vi "NNPC_Init(Train).vi"(4 "PCore_Device":T1, 6 "Dataset_Stats":T4={"means"={"R"=0.66, "G"=0.59, "B"=0.44}, "vars"={"R"=0.66, "G"=0.59, "B"=0.44}, "DS_Size"=0} {"vars"."R" format="%#_3g"; "vars"."G" format="%#_3g"; "vars"."B" format="%#_3g"; "means"."R" format="%#_3g"; "means"."G" format="%#_3g"; "means"."B" format="%#_3g"}, 7 "NN_Paths":T2={"CFG"=path "D:/Ngene/Projects_SVN/DeepLTK/R_and_D/2024_02_01_Patchcore/LabVIEW/NN_Models/PCore_L2L3_Concat_224x224/wrn/wrn_net_cfg_24_08_02__10_26_58.cfg", "BIN"=path "D:/Ngene/Projects_SVN/DeepLTK/R_and_D/2024_02_01_Patchcore/LabVIEW/NN_Models/PCore_L2L3_Concat_224x224/wrn/wrn_weights_24_08_02__10_26_58.bin"}, 8 "error in (no error)":errorcluster, 9 "Coreset_Params":T25={"Sampling_Ratio"=0.1, "Startd_idx"=3, "Random_Proj?"=TRUE, "Rnd. Proj. Params"={"Proj._Dim."=-1, "Epsilon"=0.9, "Seed"=42}}, 10 "PatchCore_Init_CFG":T23={"BackBone"=enum."WRN_50_2_L2L3", "Out_Layers_Names"=["L2", "L3"], "Patch_Size"=3}, 11 "NNFE_Custom_CFG":T28={"Input3D_Custom_Dims"={"C"=-1, "H"=-1, "W"=-1}, "mBatch"=1, "NN_Device"=enum."CPU"}) -> (0 "error out":errorcluster, 3 "PCore_Instance out":T3={"Dataset_Stats"={"means"={"R"=0.66, "G"=0.59, "B"=0.44}, "vars"={"R"=0.66, "G"=0.59, "B"=0.44}, "DS_Size"=0}, "NN"={"Name"="wrn", "No of Layers"=63, "mBatch"=1, "Layers"=[refnum, refnum, refnum, refnum, refnum, refnum, refnum, refnum, refnum, refnum, refnum, refnum, refnum, refnum, refnum, refnum, refnum, refnum, refnum, refnum, refnum, refnum, refnum, refnum, refnum, refnum, refnum, refnum, refnum, refnum, refnum, refnum, refnum, refnum, refnum, refnum, refnum, refnum, refnum, refnum, refnum, refnum, refnum, refnum, refnum, refnum, refnum, refnum, refnum, refnum, refnum, refnum, refnum, refnum, refnum, refnum, refnum, refnum, refnum, refnum, refnum, refnum, refnum], "Dimty"=enum."In3D_Out3D", "Dims_In"={"C"=3, "H"=224, "W"=224}, "Dims_Out"={"C"=302, "H"=28, "W"=28}, "Working_Dir"=path "D:/Ngene/Projects_SVN/DeepLTK/R_and_D/2024_02_01_Patchcore/LabVIEW/PatchCore_v5.0/working/wrn", "Train?"=FALSE, "Train_Params"={"Optimizer"=enum."SGD", "Beta_1"=0.999, "Beta_2"=0.999, "Weight Decay(L1)"=0.0, "Weight Decay(L2)"=0.0, "Data_Sampling"=enum."Random"}, "LR_Update_Policy"={"Policy_Type"=enum."Manual", "LR0"=0.0, "k"=0.0, "WarmUp_Policy"=enum."Step", "WarmUp_Iter"=100, "WarmUp_Ratio"=10.0}, "Session Data"={"Epochs"=0.0, "Tot_Iter"=1, "LR"=0.0, "LR_iter"=1}, "Ground_truth"={"Y"=variant(refnum<data-value> refnum)}, "NNg_hdls"={"cudnn"=2143106709504, "cublas"=2177817002560, "stream"=2141212075440, "curand"=2143055681792}, "NN_Device"=enum."GPU", "GPU Id"=0, "Labels"=["tench", "goldfish", "great white shark", "tiger shark", "hammerhead", "electric ray", "stingray", "cock", "hen", "ostrich", "brambling", "goldfinch", "house finch", "junco", "indigo bunting", "robin", "bulbul", "jay", "magpie", "chickadee", "water ouzel", "kite", "bald eagle", "vulture", "great grey owl", "European fire salamander", "common newt", "eft", "spotted salamander", "axolotl", "bullfrog", "tree frog", "tailed frog", "loggerhead", "leatherback turtle", "mud turtle", "terrapin", "box turtle", "banded gecko", "common iguana", "American chameleon", "whiptail", "agama", "frilled lizard", "alligator lizard", "Gila monster", "green lizard", "African chameleon", "Komodo dragon", "African crocodile", "American alligator", "triceratops", "thunder snake", "ringneck snake", "hognose snake", "green snake", "king snake", "garter snake", "water snake", "vine snake", "night snake", "boa constrictor", "rock python", "Indian cobra", "green mamba", "sea snake", "horned viper", "diamondback", "sidewinder", "trilobite", "harvestman", "scorpion", "black and gold garden spider", "barn spider", "garden spider", "black widow", "tarantula", "wolf spider", "tick", "centipede", "black grouse", "ptarmigan", "ruffed grouse", "prairie chicken", "peacock", "quail", "partridge", "African grey", "macaw", "sulphur-crested cockatoo", "lorikeet", "coucal", "bee eater", "hornbill", "hummingbird", "jacamar", "toucan", "drake", "red-breasted merganser", "goose", "black swan", "tusker", "echidna", "platypus", "wallaby", "koala", "wombat", "jellyfish", "sea anemone", "brain coral", "flatworm", "nematode", "conch", "snail", "slug", "sea slug", "chiton", "chambered nautilus", "Dungeness crab", "rock crab", "fiddler crab", "king crab", "American lobster", "spiny lobster", "crayfish", "hermit crab", "isopod", "white stork", "black stork", "spoonbill", "flamingo", "little blue heron", "American egret", "bittern", "crane", "limpkin", "European gallinule", "American coot", "bustard", "ruddy turnstone", "red-backed sandpiper", "redshank", "dowitcher", "oystercatcher", "pelican", "king penguin", "albatross", "grey whale", "killer whale", "dugong", "sea lion", "Chihuahua", "Japanese spaniel", "Maltese dog", "Pekinese", "Shih-Tzu", "Blenheim spaniel", "papillon", "toy terrier", "Rhodesian ridgeback", "Afghan hound", "basset", "beagle", "bloodhound", "bluetick", "black-and-tan coonhound", "Walker hound", "English foxhound", "redbone", "borzoi", "Irish wolfhound", "Italian greyhound", "whippet", "Ibizan hound", "Norwegian elkhound", "otterhound", "Saluki", "Scottish deerhound", "Weimaraner", "Staffordshire bullterrier", "American Staffordshire terrier", "Bedlington terrier", "Border terrier", "Kerry blue terrier", "Irish terrier", "Norfolk terrier", "Norwich terrier", "Yorkshire terrier", "wire-haired fox terrier", "Lakeland terrier", "Sealyham terrier", "Airedale", "cairn", "Australian terrier", "Dandie Dinmont", "Boston bull", "miniature schnauzer", "giant schnauzer", "standard schnauzer", "Scotch terrier", "Tibetan terrier", "silky terrier", "soft-coated wheaten terrier", "West Highland white terrier", "Lhasa", "flat-coated retriever", "curly-coated retriever", "golden retriever", "Labrador retriever", "Chesapeake Bay retriever", "German short-haired pointer", "vizsla", "English setter", "Irish setter", "Gordon setter", "Brittany spaniel", "clumber", "English springer", "Welsh springer spaniel", "cocker spaniel", "Sussex spaniel", "Irish water spaniel", "kuvasz", "schipperke", "groenendael", "malinois", "briard", "kelpie", "komondor", "Old English sheepdog", "Shetland sheepdog", "collie", "Border collie", "Bouvier des Flandres", "Rottweiler", "German shepherd", "Doberman", "miniature pinscher", "Greater Swiss Mountain dog", "Bernese mountain dog", "Appenzeller", "EntleBucher", "boxer", "bull mastiff", "Tibetan mastiff", "French bulldog", "Great Dane", "Saint Bernard", "Eskimo dog", "malamute", "Siberian husky", "dalmatian", "affenpinscher", "basenji", "pug", "Leonberg", "Newfoundland", "Great Pyrenees", "Samoyed", "Pomeranian", "chow", "keeshond", "Brabancon griffon", "Pembroke", "Cardigan", "toy poodle", "miniature poodle", "standard poodle", "Mexican hairless", "timber wolf", "white wolf", "red wolf", "coyote", "dingo", "dhole", "African hunting dog", "hyena", "red fox", "kit fox", "Arctic fox", "grey fox", "tabby", "tiger cat", "Persian cat", "Siamese cat", "Egyptian cat", "cougar", "lynx", "leopard", "snow leopard", "jaguar", "lion", "tiger", "cheetah", "brown bear", "American black bear", "ice bear", "sloth bear", "mongoose", "meerkat", "tiger beetle", "ladybug", "ground beetle", "long-horned beetle", "leaf beetle", "dung beetle", "rhinoceros beetle", "weevil", "fly", "bee", "ant", "grasshopper", "cricket", "walking stick", "cockroach", "mantis", "cicada", "leafhopper", "lacewing", "dragonfly", "damselfly", "admiral", "ringlet", "monarch", "cabbage butterfly", "sulphur butterfly", "lycaenid", "starfish", "sea urchin", "sea cucumber", "wood rabbit", "hare", "Angora", "hamster", "porcupine", "fox squirrel", "marmot", "beaver", "guinea pig", "sorrel", "zebra", "hog", "wild boar", "warthog", "hippopotamus", "ox", "water buffalo", "bison", "ram", "bighorn", "ibex", "hartebeest", "impala", "gazelle", "Arabian camel", "llama", "weasel", "mink", "polecat", "black-footed ferret", "otter", "skunk", "badger", "armadillo", "three-toed sloth", "orangutan", "gorilla", "chimpanzee", "gibbon", "siamang", "guenon", "patas", "baboon", "macaque", "langur", "colobus", "proboscis monkey", "marmoset", "capuchin", "howler monkey", "titi", "spider monkey", "squirrel monkey", "Madagascar cat", "indri", "Indian elephant", "African elephant", "lesser panda", "giant panda", "barracouta", "eel", "coho", "rock beauty", "anemone fish", "sturgeon", "gar", "lionfish", "puffer", "abacus", "abaya", "academic gown", "accordion", "acoustic guitar", "aircraft carrier", "airliner", "airship", "altar", "ambulance", "amphibian", "analog clock", "apiary", "apron", "ashcan", "assault rifle", "backpack", "bakery", "balance beam", "balloon", "ballpoint", "Band Aid", "banjo", "bannister", "barbell", "barber chair", "barbershop", "barn", "barometer", "barrel", "barrow", "baseball", "basketball", "bassinet", "bassoon", "bathing cap", "bath towel", "bathtub", "beach wagon", "beacon", "beaker", "bearskin", "beer bottle", "beer glass", "bell cote", "bib", "bicycle-built-for-two", "bikini", "binder", "binoculars", "birdhouse", "boathouse", "bobsled", "bolo tie", "bonnet", "bookcase", "bookshop", "bottlecap", "bow", "bow tie", "brass", "brassiere", "breakwater", "breastplate", "broom", "bucket", "buckle", "bulletproof vest", "bullet train", "butcher shop", "cab", "caldron", "candle", "cannon", "canoe", "can opener", "cardigan", "car mirror", "carousel", "carpenter's kit", "carton", "car wheel", "cash machine", "cassette", "cassette player", "castle", "catamaran", "CD player", "cello", "cellular telephone", "chain", "chainlink fence", "chain mail", "chain saw", "chest", "chiffonier", "chime", "china cabinet", "Christmas stocking", "church", "cinema", "cleaver", "cliff dwelling", "cloak", "clog", "cocktail shaker", "coffee mug", "coffeepot", "coil", "combination lock", "computer keyboard", "confectionery", "container ship", "convertible", "corkscrew", "cornet", "cowboy boot", "cowboy hat", "cradle", "crane", "crash helmet", "crate", "crib", "Crock Pot", "croquet ball", "crutch", "cuirass", "dam", "desk", "desktop computer", "dial telephone", "diaper", "digital clock", "digital watch", "dining table", "dishrag", "dishwasher", "disk brake", "dock", "dogsled", "dome", "doormat", "drilling platform", "drum", "drumstick", "dumbbell", "Dutch oven", "electric fan", "electric guitar", "electric locomotive", "entertainment center", "envelope", "espresso maker", "face powder", "feather boa", "file", "fireboat", "fire engine", "fire screen", "flagpole", "flute", "folding chair", "football helmet", "forklift", "fountain", "fountain pen", "four-poster", "freight car", "French horn", "frying pan", "fur coat", "garbage truck", "gasmask", "gas pump", "goblet", "go-kart", "golf ball", "golfcart", "gondola", "gong", "gown", "grand piano", "greenhouse", "grille", "grocery store", "guillotine", "hair slide", "hair spray", "half track", "hammer", "hamper", "hand blower", "hand-held computer", "handkerchief", "hard disc", "harmonica", "harp", "harvester", "hatchet", "holster", "home theater", "honeycomb", "hook", "hoopskirt", "horizontal bar", "horse cart", "hourglass", "iPod", "iron", "jack-o'-lantern", "jean", "jeep", "jersey", "jigsaw puzzle", "jinrikisha", "joystick", "kimono", "knee pad", "knot", "lab coat", "ladle", "lampshade", "laptop", "lawn mower", "lens cap", "letter opener", "library", "lifeboat", "lighter", "limousine", "liner", "lipstick", "Loafer", "lotion", "loudspeaker", "loupe", "lumbermill", "magnetic compass", "mailbag", "mailbox", "maillot", "maillot", "manhole cover", "maraca", "marimba", "mask", "matchstick", "maypole", "maze", "measuring cup", "medicine chest", "megalith", "microphone", "microwave", "military uniform", "milk can", "minibus", "miniskirt", "minivan", "missile", "mitten", "mixing bowl", "mobile home", "Model T", "modem", "monastery", "monitor", "moped", "mortar", "mortarboard", "mosque", "mosquito net", "motor scooter", "mountain bike", "mountain tent", "mouse", "mousetrap", "moving van", "muzzle", "nail", "neck brace", "necklace", "nipple", "notebook", "obelisk", "oboe", "ocarina", "odometer", "oil filter", "organ", "oscilloscope", "overskirt", "oxcart", "oxygen mask", "packet", "paddle", "paddlewheel", "padlock", "paintbrush", "pajama", "palace", "panpipe", "paper towel", "parachute", "parallel bars", "park bench", "parking meter", "passenger car", "patio", "pay-phone", "pedestal", "pencil box", "pencil sharpener", "perfume", "Petri dish", "photocopier", "pick", "pickelhaube", "picket fence", "pickup", "pier", "piggy bank", "pill bottle", "pillow", "ping-pong ball", "pinwheel", "pirate", "pitcher", "plane", "planetarium", "plastic bag", "plate rack", "plow", "plunger", "Polaroid camera", "pole", "police van", "poncho", "pool table", "pop bottle", "pot", "potter's wheel", "power drill", "prayer rug", "printer", "prison", "projectile", "projector", "puck", "punching bag", "purse", "quill", "quilt", "racer", "racket", "radiator", "radio", "radio telescope", "rain barrel", "recreational vehicle", "reel", "reflex camera", "refrigerator", "remote control", "restaurant", "revolver", "rifle", "rocking chair", "rotisserie", "rubber eraser", "rugby ball", "rule", "running shoe", "safe", "safety pin", "saltshaker", "sandal", "sarong", "sax", "scabbard", "scale", "school bus", "schooner", "scoreboard", "screen", "screw", "screwdriver", "seat belt", "sewing machine", "shield", "shoe shop", "shoji", "shopping basket", "shopping cart", "shovel", "shower cap", "shower curtain", "ski", "ski mask", "sleeping bag", "slide rule", "sliding door", "slot", "snorkel", "snowmobile", "snowplow", "soap dispenser", "soccer ball", "sock", "solar dish", "sombrero", "soup bowl", "space bar", "space heater", "space shuttle", "spatula", "speedboat", "spider web", "spindle", "sports car", "spotlight", "stage", "steam locomotive", "steel arch bridge", "steel drum", "stethoscope", "stole", "stone wall", "stopwatch", "stove", "strainer", "streetcar", "stretcher", "studio couch", "stupa", "submarine", "suit", "sundial", "sunglass", "sunglasses", "sunscreen", "suspension bridge", "swab", "sweatshirt", "swimming trunks", "swing", "switch", "syringe", "table lamp", "tank", "tape player", "teapot", "teddy", "television", "tennis ball", "thatch", "theater curtain", "thimble", "thresher", "throne", "tile roof", "toaster", "tobacco shop", "toilet seat", "torch", "totem pole", "tow truck", "toyshop", "tractor", "trailer truck", "tray", "trench coat", "tricycle", "trimaran", "tripod", "triumphal arch", "trolleybus", "trombone", "tub", "turnstile", "typewriter keyboard", "umbrella", "unicycle", "upright", "vacuum", "vase", "vault", "velvet", "vending machine", "vestment", "viaduct", "violin", "volleyball", "waffle iron", "wall clock", "wallet", "wardrobe", "warplane", "washbasin", "washer", "water bottle", "water jug", "water tower", "whiskey jug", "whistle", "wig", "window screen", "window shade", "Windsor tie", "wine bottle", "wing", "wok", "wooden spoon", "wool", "worm fence", "wreck", "yawl", "yurt", "web site", "comic book", "crossword puzzle", "street sign", "traffic light", "book jacket", "menu", "plate", "guacamole", "consomme", "hot pot", "trifle", "ice cream", "ice lolly", "French loaf", "bagel", "pretzel", "cheeseburger", "hotdog", "mashed potato", "head cabbage", "broccoli", "cauliflower", "zucchini", "spaghetti squash", "acorn squash", "butternut squash", "cucumber", "artichoke", "bell pepper", "cardoon", "mushroom", "Granny Smith", "strawberry", "orange", "lemon", "fig", "pineapple", "banana", "jackfruit", "custard apple", "pomegranate", "hay", "carbonara", "chocolate sauce", "dough", "meat loaf", "pizza", "potpie", "burrito", "red wine", "espresso", "cup", "eggnog", "alp", "bubble", "cliff", "coral reef", "geyser", "lakeside", "promontory", "sandbar", "seashore", "valley", "volcano", "ballplayer", "groom", "scuba diver", "rapeseed", "daisy", "yellow lady's slipper", "corn", "acorn", "hip", "buckeye", "coral fungus", "agaric", "gyromitra", "stinkhorn", "earthstar", "hen-of-the-woods", "bolete", "ear", "toilet tissue"], "Receptive Field"=[{"V"=1, "H"=1}, {"V"=7, "H"=7}, {"V"=9, "H"=9}, {"V"=9, "H"=9}, {"V"=21, "H"=21}, {"V"=21, "H"=21}, {"V"=9, "H"=9}, {"V"=21, "H"=21}, {"V"=21, "H"=21}, {"V"=33, "H"=33}, {"V"=33, "H"=33}, {"V"=33, "H"=33}, {"V"=33, "H"=33}, {"V"=45, "H"=45}, {"V"=45, "H"=45}, {"V"=45, "H"=45}, {"V"=45, "H"=45}, {"V"=57, "H"=57}, {"V"=57, "H"=57}, {"V"=45, "H"=45}, {"V"=57, "H"=57}, {"V"=57, "H"=57}, {"V"=81, "H"=81}, {"V"=81, "H"=81}, {"V"=81, "H"=81}, {"V"=81, "H"=81}, {"V"=105, "H"=105}, {"V"=105, "H"=105}, {"V"=105, "H"=105}, {"V"=105, "H"=105}, {"V"=129, "H"=129}, {"V"=129, "H"=129}, {"V"=129, "H"=129}, {"V"=129, "H"=129}, {"V"=153, "H"=153}, {"V"=153, "H"=153}, {"V"=129, "H"=129}, {"V"=153, "H"=153}, {"V"=153, "H"=153}, {"V"=201, "H"=201}, {"V"=201, "H"=201}, {"V"=201, "H"=201}, {"V"=201, "H"=201}, {"V"=249, "H"=249}, {"V"=249, "H"=249}, {"V"=249, "H"=249}, {"V"=249, "H"=249}, {"V"=297, "H"=297}, {"V"=297, "H"=297}, {"V"=297, "H"=297}, {"V"=297, "H"=297}, {"V"=345, "H"=345}, {"V"=345, "H"=345}, {"V"=345, "H"=345}, {"V"=345, "H"=345}, {"V"=393, "H"=393}, {"V"=393, "H"=393}, {"V"=393, "H"=393}, {"V"=153, "H"=153}, {"V"=441, "H"=441}, {"V"=441, "H"=441}, {"V"=441, "H"=441}, {"V"=441, "H"=441}], "Loss_Type"=enum."MSE", "Loss_Cfg_Prms"=variant, "NNG_WS"={"NNG_WS_Mem"=refnum, "Max_WS_Size"=-1}}, "PCore_Device"=enum."GPU(CuLab)", "PatchCore_Init_CFG"={"BackBone"=enum."WRN_50_2_L2L3", "Out_Layers_Names"=[], "Patch_Size"=0}, "Coreset Params"={"Sampling_Ratio"=0.0, "Startd_idx"=0, "Random_Proj?"=FALSE, "Rnd. Proj. Params"={"Proj._Dim."=0, "Epsilon"=0.9, "Seed"=42}}, "MemBank_Data"={"MemBank"=variant, "MemBank Norm"=variant}} {"NN out"."LR_Update_Policy"."WarmUp_Ratio" min=1; "NN out"."LR_Update_Policy"."WarmUp_Iter" min=1; "NN out"."LR_Update_Policy"."LR0" format="%.7f"; "Dataset_Stats"."vars"."R" format="%#_3g"; "Dataset_Stats"."vars"."G" format="%#_3g"; "Dataset_Stats"."vars"."B" format="%#_3g"; "Dataset_Stats"."means"."R" format="%#_3g"; "Dataset_Stats"."means"."G" format="%#_3g"; "Dataset_Stats"."means"."B" format="%#_3g"}, 5 "dT":dbl)   [LabVIEW 2020]
uses:
  Controls/PatchCore_Init_CFG.ctl
  Controls/PatchCore_BackBone_Selector.ctl
  Controls/PatchCore_Init_Custom_NN_CFG.ctl
  <vilib>/Ngene/Deep Learning Toolkit/Toolkit/NN_Data/API/NN_Dims(C,H,W).ctl
  <vilib>/Ngene/Deep Learning Toolkit/Toolkit/NN_Network/Controls/NN_Device.ctl
  Controls/PatchCore_DS_Stats.ctl
  Controls/Image_Stats_RGB.ctl
  Controls/Coreset_Params.ctl
  Controls/Random_Projection_Coreset.ctl
  Controls/PatchCore_Instance.ctl
  <vilib>/Ngene/Deep Learning Toolkit/Toolkit/NN_Network/Controls/NN.ctl
  <vilib>/Ngene/Deep Learning Toolkit/Toolkit/NN_Layers/Controls/NN_Layer_ref.ctl
  <vilib>/Ngene/Deep Learning Toolkit/Toolkit/NN_Layers/Controls/NN_Layer.ctl
  <vilib>/Ngene/Deep Learning Toolkit/Toolkit/NN_Layers/Controls/NN_Layer_Type.ctl
  <vilib>/Ngene/Deep Learning Toolkit/Toolkit/NN_Layers/Controls/NN_Layer_Metrics.ctl
  <vilib>/Ngene/Deep Learning Toolkit/Toolkit/NNg/cuda/Controls/nng_cuda_handles.ctl
  <vilib>/Ngene/Deep Learning Toolkit/Toolkit/NN_Layers/Controls/NN_Layer_Dimty.ctl
  <vilib>/Ngene/Deep Learning Toolkit/Toolkit/NN_Layers/Controls/NN_Layer_RF_State.ctl
  <vilib>/Ngene/Deep Learning Toolkit/Toolkit/NN_Data/API/NN_Dims(V,H).ctl
  <vilib>/Ngene/Deep Learning Toolkit/Toolkit/NN_Network/Controls/NN_In_Out_Dim-ty.ctl
  <vilib>/Ngene/Deep Learning Toolkit/Toolkit/NN_Train/Controls/NN_Train_Params.ctl
  <vilib>/Ngene/Deep Learning Toolkit/Toolkit/NN_Train/Controls/NN_Train_Optimizer.ctl
  <vilib>/Ngene/Deep Learning Toolkit/Toolkit/NN_Train/Controls/NN_Train_Data_Sampling.ctl
  <vilib>/Ngene/Deep Learning Toolkit/Toolkit/NN_Train/Controls/NN_LR_Policy_Cfg.ctl
  <vilib>/Ngene/Deep Learning Toolkit/Toolkit/NN_Train/Controls/NN_LR_Policy_Type.ctl
  <vilib>/Ngene/Deep Learning Toolkit/Toolkit/NN_Train/Controls/NN_Train_Session_Data.ctl
  <vilib>/Ngene/Deep Learning Toolkit/Toolkit/NN_Data/Controls/NN_Ground_truth.ctl
  <vilib>/Ngene/Deep Learning Toolkit/Toolkit/NN_Train/Controls/NN_Loss_Type.ctl
  <vilib>/Ngene/Deep Learning Toolkit/Toolkit/NNg/Network/WS/Controls/NNG_WS.ctl
  <vilib>/Ngene/Deep Learning Toolkit/Toolkit/NNg/Network/WS/Controls/NNg_WS_Mem_DVR.ctl
  <vilib>/Ngene/Deep Learning Toolkit/Toolkit/NNg/cuda/Controls/cuda_Mem_desc.ctl
  Controls/PCore_Device.ctl
  Controls/MemBank_and_Norm_Variants.ctl
  Controls/NN_Paths.ctl
  edddb0eb-9e83-41dd-b3bf-18adf70eff0a.vi
  e3f785a9-3252-4081-a6fc-ec5b49997386.vi
  <vilib>/Utility/High Resolution Relative Seconds.vi
  <vilib>/Ngene/Deep Learning Toolkit/Toolkit/Deep_Learning_Toolkit_by_Ngene.lvlib
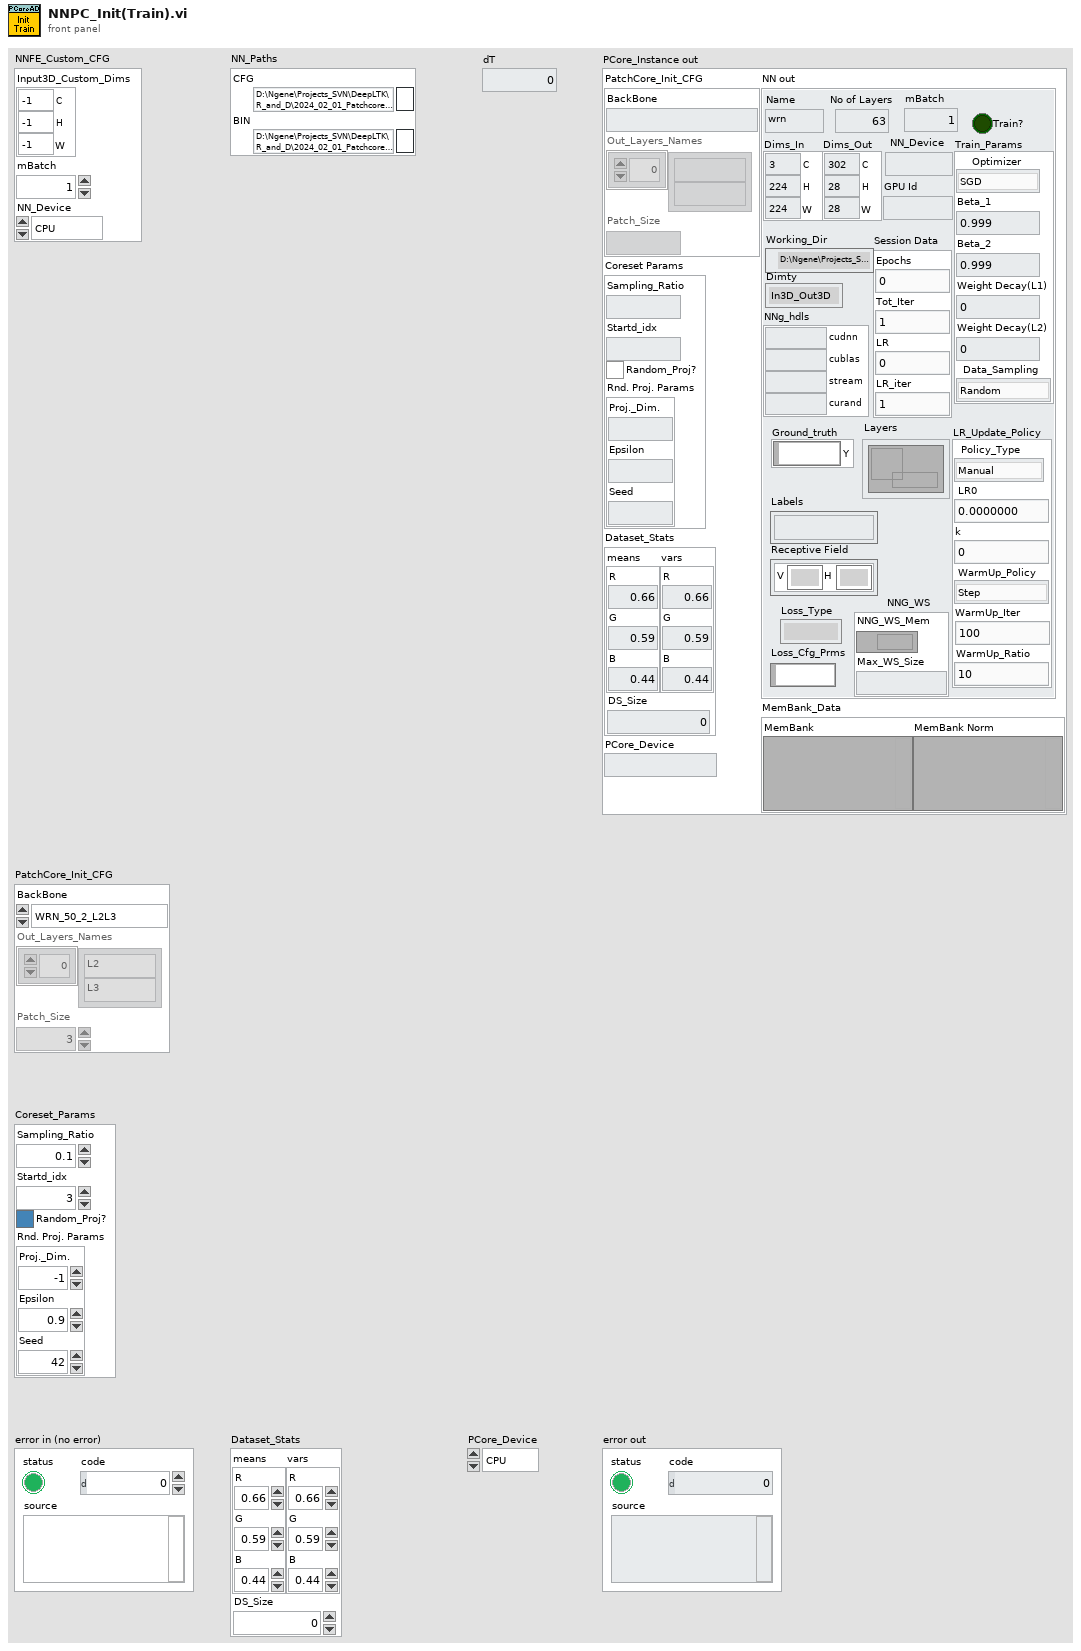
[diagram p1: front panel]
types:
  T1 = typedef "PCore_Device.ctl" = enum16{"CPU", "GPU(CuLab)"}
  T2 = typedef "NN_Paths.ctl" = cluster{"CFG":path, "BIN":path}
  T3 = typedef "PatchCore_Instance.ctl" = cluster{"Dataset_Stats":T4, "NN":T6, "PCore_Device":T1, "PatchCore_Init_CFG":T23, "Coreset Params":T25, "MemBank_Data":T27}
  T4 = typedef "PatchCore_DS_Stats.ctl" = cluster{"means":T5, "vars":T5, "DS_Size":i32}
  T5 = typedef "Image_Stats_RGB.ctl" = cluster{"R":sgl, "G":sgl, "B":sgl}
  T6 = typedef "Deep_Learning_Toolkit_by_Ngene.lvlib/NN.ctl" = cluster{"Name":string, "No of Layers":i32, "mBatch":i32, "Layers":T7[], "Dimty":T8, "Dims_In":T9, "Dims_Out":T9, "Working_Dir":path, "Train?":bool, "Train_Params":T10, "LR_Update_Policy":T13, "Session Data":T15, "Ground_truth":T16, "NNg_hdls":T17, "NN_Device":T18, "GPU Id":i32, "Labels":string[], "Receptive Field":T19[], "Loss_Type":T20, "Loss_Cfg_Prms":variant, "NNG_WS":T21}
  T7 = typedef "Deep_Learning_Toolkit_by_Ngene.lvlib/NN_Layer_ref.ctl" = refnum<data-value>
  T8 = typedef "Deep_Learning_Toolkit_by_Ngene.lvlib/NN_In_Out_Dim-ty.ctl" = enum8{"In1D_Out1D", "In3D_Out1D", "In3D_Out3D", "In3D_OutBBox"}
  T9 = typedef "Deep_Learning_Toolkit_by_Ngene.lvlib/NN_Dims(C,H,W).ctl" = cluster{"C":i32, "H":i32, "W":i32}
  T10 = typedef "Deep_Learning_Toolkit_by_Ngene.lvlib/NN_Train_Params.ctl" = cluster{"Optimizer":T11, "Beta_1":sgl, "Beta_2":sgl, "Weight Decay(L1)":sgl, "Weight Decay(L2)":sgl, "Data_Sampling":T12}
  T11 = typedef "Deep_Learning_Toolkit_by_Ngene.lvlib/NN_Train_Optimizer.ctl" = enum16{"SGD", "Adam", "Adagrad", "Adadelta", "RMSProp", "Nesterov"}
  T12 = typedef "Deep_Learning_Toolkit_by_Ngene.lvlib/NN_Train_Data_Sampling.ctl" = enum16{"Random", "Sequential"}
  T13 = typedef "Deep_Learning_Toolkit_by_Ngene.lvlib/NN_LR_Policy_Cfg.ctl" = cluster{"Policy_Type":T14, "LR0":dbl, "k":sgl, "WarmUp_Policy":enum16{"Step", "Ramp"}, "WarmUp_Iter":i32, "WarmUp_Ratio":sgl}
  T14 = typedef "Deep_Learning_Toolkit_by_Ngene.lvlib/NN_LR_Policy_Type.ctl" = enum16{"Manual", "Step", "Exp", "1/t"}
  T15 = typedef "Deep_Learning_Toolkit_by_Ngene.lvlib/NN_Train_Session_Data.ctl" = cluster{"Epochs":sgl, "Tot_Iter":i32, "LR":sgl, "LR_iter":i32}
  T16 = typedef "Deep_Learning_Toolkit_by_Ngene.lvlib/NN_Ground_truth.ctl" = cluster{"Y":variant}
  T17 = typedef "Deep_Learning_Toolkit_by_Ngene.lvlib/nng_cuda_handles.ctl" = cluster{"cudnn":u64, "cublas":u64, "stream":u64, "curand":u64}
  T18 = typedef "Deep_Learning_Toolkit_by_Ngene.lvlib/NN_Device.ctl" = enum16{"CPU", "GPU"}
  T19 = typedef "Deep_Learning_Toolkit_by_Ngene.lvlib/NN_Dims(V,H).ctl" = cluster{"V":i32, "H":i32}
  T20 = typedef "Deep_Learning_Toolkit_by_Ngene.lvlib/NN_Loss_Type.ctl" = enum16{"None", "MSE", "CrossEntropy", "YOLO_v2", "YOLO_v4"}
  T21 = typedef "Deep_Learning_Toolkit_by_Ngene.lvlib/NNG_WS.ctl" = cluster{"NNG_WS_Mem":T22, "Max_WS_Size":i64}
  T22 = typedef "Deep_Learning_Toolkit_by_Ngene.lvlib/NNg_WS_Mem_DVR.ctl" = refnum<data-value>
  T23 = typedef "PatchCore_Init_CFG.ctl" = cluster{"BackBone":T24, "Out_Layers_Names":string[], "Patch_Size":u32}
  T24 = typedef "PatchCore_BackBone_Selector.ctl" = enum16{"WRN_50_2_L2L3"}
  T25 = typedef "Coreset_Params.ctl" = cluster{"Sampling_Ratio":sgl, "Startd_idx":i32, "Random_Proj?":bool, "Rnd. Proj. Params":T26}
  T26 = typedef "Random_Projection_Coreset.ctl" = cluster{"Proj._Dim.":i32, "Epsilon":sgl, "Seed":i32}
  T27 = typedef "MemBank_and_Norm_Variants.ctl" = cluster{"MemBank":variant, "MemBank Norm":variant}
  T28 = typedef "PatchCore_Init_Custom_NN_CFG.ctl" = cluster{"Input3D_Custom_Dims":T9, "mBatch":i32, "NN_Device":T18}
  T29 = typedef "Deep_Learning_Toolkit_by_Ngene.lvlib/NN_Config_Params.ctl" = cluster{"Name":string, "mBatch":i32, "NN_Train_Params":T10, "LR_Decay_Policy":T13, "Labels":string[], "Loss":T30}
  T30 = typedef "Deep_Learning_Toolkit_by_Ngene.lvlib/NN_Loss_Config_Params.ctl" = cluster{"Loss_Type":T20, "Loss_Conf_Params":variant}
  T31 = typedef "Deep_Learning_Toolkit_by_Ngene.lvlib/NN_Layer_Config_Params.ctl" = cluster{"Layer_Type":T32, "Layer_Conf_Params":variant, "Input Layers":string[]}
  T32 = typedef "Deep_Learning_Toolkit_by_Ngene.lvlib/NN_Layer_Type.ctl" = enum16{"Input1D", "Input3D", "Conv1D", "Conv2D", "Conv2D_Adv", "MaxPool", "AvgPool", "UpSample", "DropOut3D", "ShortCut", "Concat", "SoftMax3D", "FC", "DropOut", "Softmax", "Flatten", "YOLO_v2", "YOLO_v4", "Activation", "BatchNormalization", "Unsupported"}
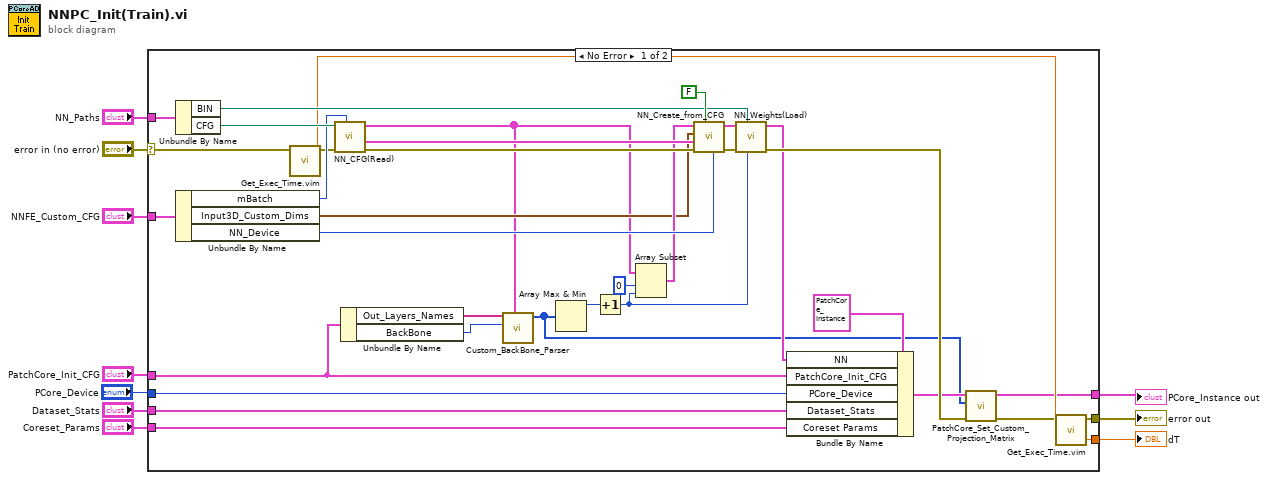
[diagram p0: block diagram]
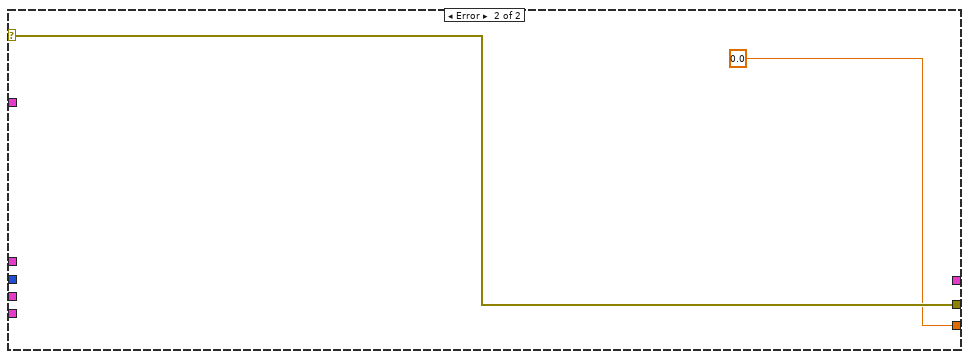
[diagram p2: hidden frame]
diagram:
  n1 = case shown="No Error" "error in (no error)" {
    selector: "error in (no error)" -> [w29 w47]
    tunnel: "PatchCore_Init_CFG" -> [w13 _]
    tunnel: "NN_Paths" -> [w41 _]
    tunnel: "NNFE_Custom_CFG" -> [w38 _]
    tunnel: "Dataset_Stats" -> [w31 _]
    tunnel: [w27 w47] -> w7
    tunnel: [w26 0.0 ("dT")] -> w6
    tunnel: [w19 _] -> w3
    tunnel: "Coreset_Params" -> [w12 _]
    tunnel: "PCore_Device" -> [w14 _]
    frame No Error {
      n2 = Unbundle By Name(w41) -> ("BIN"=w37:path, "CFG"=w40:path)
      n3 = Unbundle By Name(w38) -> ("mBatch"=w36:i32, "Input3D_Custom_Dims"=w23:T9, "NN_Device"=w39:T18)
      n4 = call "Get_Exec_Time.vim"("error in (no error)"=w29) -> ("T(n)"=w24:dbl, "error out"=w28:errorcluster)  [unwired: 6 in, 1 out]
      n5 = call <vilib>:"NN_CFG(Read).vi"("mBatch"=w36, "error in (no error)"=w28, "CFG file path"=w40) -> ("error out"=w43:errorcluster, "Net_Cfg"=w44:T29, "Layer_Cfg"=w16:T31[])  [unwired: 6 in]
      n6 = Unbundle By Name(w13) -> ("Out_Layers_Names"=w25:string[], "BackBone"=w22:T24)
      n7 = call "Custom_BackBone_Parser.vi"("Layer_Cfg"=w16, "BackBone"=w22, "Out_Layers_Names"=w25) -> ("Out_Layers_Idx"=w11:i32[])  [unwired: 8 in]
      n8 = Array Max & Min(array=w11) -> (max value=w33:i32)  [unwired: 3 out]
      n9 = Increment(x=w33) -> (x+1=w32:i32)
      n10 = Array Subset(array=w16, index=0, length=w32) -> (w34:T31[])
      n11 = call <vilib>:"NN_Create_from_CFG.vi"("NN_Device"=w39, "Train? (false)"=FALSE, "error in (no error)"=w43, "Net_Cfg"=w44, "Input3D_Custom_Dims"=w23, "Layer_Cfg"=w34) -> ("error out"=w42:errorcluster, "NN out"=w30:T6)  [unwired: 4 in]
      n12 = call <vilib>:"NN_Weights(Load).vi"("Up To"=w32, "Weight File Path"=w37, "error in (no error)"=w42, "NN in"=w30) -> ("error out"=w21:errorcluster, "NN out"=w18:T6)  [unwired: 6 in]
      n13 = Bundle By Name(cluster=T3 {"Dataset_Stats"={"means"={"R"=0.66, "G"=0.59, "B"=0.44}, "vars"={"R"=0.66, "G"=0.59, "B"=0.44}, "DS_Size"=0}, "NN"={"Name"="wrn", "No of Layers"=63, "mBatch"=1, "Layers"=[refnum, refnum, refnum, refnum, refnum, refnum, refnum, refnum, refnum, refnum, refnum, refnum, refnum, refnum, refnum, refnum, refnum, refnum, refnum, refnum, refnum, refnum, refnum, refnum, refnum, refnum, refnum, refnum, refnum, refnum, refnum, refnum, refnum, refnum, refnum, refnum, refnum, refnum, refnum, refnum, refnum, refnum, refnum, refnum, refnum, refnum, refnum, refnum, refnum, refnum, refnum, refnum, refnum, refnum, refnum, refnum, refnum, refnum, refnum, refnum, refnum, refnum, refnum], "Dimty"=enum."In3D_Out3D", "Dims_In"={"C"=3, "H"=224, "W"=224}, "Dims_Out"={"C"=302, "H"=28, "W"=28}, "Working_Dir"=path "D:/Ngene/Projects_SVN/DeepLTK/R_and_D/2024_02_01_Patchcore/LabVIEW/PatchCore_v5.0/working/wrn", "Train?"=FALSE, "Train_Params"={"Optimizer"=enum."SGD", "Beta_1"=0.999, "Beta_2"=0.999, "Weight Decay(L1)"=0.0, "Weight Decay(L2)"=0.0, "Data_Sampling"=enum."Random"}, "LR_Update_Policy"={"Policy_Type"=enum."Manual", "LR0"=0.0, "k"=0.0, "WarmUp_Policy"=enum."Step", "WarmUp_Iter"=100, "WarmUp_Ratio"=10.0}, "Session Data"={"Epochs"=0.0, "Tot_Iter"=1, "LR"=0.0, "LR_iter"=1}, "Ground_truth"={"Y"=variant(refnum<data-value> refnum)}, "NNg_hdls"={"cudnn"=2143106709504, "cublas"=2177817002560, "stream"=2141212075440, "curand"=2143055681792}, "NN_Device"=enum."GPU", "GPU Id"=0, "Labels"=["tench", "goldfish", "great white shark", "tiger shark", "hammerhead", "electric ray", "stingray", "cock", "hen", "ostrich", "brambling", "goldfinch", "house finch", "junco", "indigo bunting", "robin", "bulbul", "jay", "magpie", "chickadee", "water ouzel", "kite", "bald eagle", "vulture", "great grey owl", "European fire salamander", "common newt", "eft", "spotted salamander", "axolotl", "bullfrog", "tree frog", "tailed frog", "loggerhead", "leatherback turtle", "mud turtle", "terrapin", "box turtle", "banded gecko", "common iguana", "American chameleon", "whiptail", "agama", "frilled lizard", "alligator lizard", "Gila monster", "green lizard", "African chameleon", "Komodo dragon", "African crocodile", "American alligator", "triceratops", "thunder snake", "ringneck snake", "hognose snake", "green snake", "king snake", "garter snake", "water snake", "vine snake", "night snake", "boa constrictor", "rock python", "Indian cobra", "green mamba", "sea snake", "horned viper", "diamondback", "sidewinder", "trilobite", "harvestman", "scorpion", "black and gold garden spider", "barn spider", "garden spider", "black widow", "tarantula", "wolf spider", "tick", "centipede", "black grouse", "ptarmigan", "ruffed grouse", "prairie chicken", "peacock", "quail", "partridge", "African grey", "macaw", "sulphur-crested cockatoo", "lorikeet", "coucal", "bee eater", "hornbill", "hummingbird", "jacamar", "toucan", "drake", "red-breasted merganser", "goose", "black swan", "tusker", "echidna", "platypus", "wallaby", "koala", "wombat", "jellyfish", "sea anemone", "brain coral", "flatworm", "nematode", "conch", "snail", "slug", "sea slug", "chiton", "chambered nautilus", "Dungeness crab", "rock crab", "fiddler crab", "king crab", "American lobster", "spiny lobster", "crayfish", "hermit crab", "isopod", "white stork", "black stork", "spoonbill", "flamingo", "little blue heron", "American egret", "bittern", "crane", "limpkin", "European gallinule", "American coot", "bustard", "ruddy turnstone", "red-backed sandpiper", "redshank", "dowitcher", "oystercatcher", "pelican", "king penguin", "albatross", "grey whale", "killer whale", "dugong", "sea lion", "Chihuahua", "Japanese spaniel", "Maltese dog", "Pekinese", "Shih-Tzu", "Blenheim spaniel", "papillon", "toy terrier", "Rhodesian ridgeback", "Afghan hound", "basset", "beagle", "bloodhound", "bluetick", "black-and-tan coonhound", "Walker hound", "English foxhound", "redbone", "borzoi", "Irish wolfhound", "Italian greyhound", "whippet", "Ibizan hound", "Norwegian elkhound", "otterhound", "Saluki", "Scottish deerhound", "Weimaraner", "Staffordshire bullterrier", "American Staffordshire terrier", "Bedlington terrier", "Border terrier", "Kerry blue terrier", "Irish terrier", "Norfolk terrier", "Norwich terrier", "Yorkshire terrier", "wire-haired fox terrier", "Lakeland terrier", "Sealyham terrier", "Airedale", "cairn", "Australian terrier", "Dandie Dinmont", "Boston bull", "miniature schnauzer", "giant schnauzer", "standard schnauzer", "Scotch terrier", "Tibetan terrier", "silky terrier", "soft-coated wheaten terrier", "West Highland white terrier", "Lhasa", "flat-coated retriever", "curly-coated retriever", "golden retriever", "Labrador retriever", "Chesapeake Bay retriever", "German short-haired pointer", "vizsla", "English setter", "Irish setter", "Gordon setter", "Brittany spaniel", "clumber", "English springer", "Welsh springer spaniel", "cocker spaniel", "Sussex spaniel", "Irish water spaniel", "kuvasz", "schipperke", "groenendael", "malinois", "briard", "kelpie", "komondor", "Old English sheepdog", "Shetland sheepdog", "collie", "Border collie", "Bouvier des Flandres", "Rottweiler", "German shepherd", "Doberman", "miniature pinscher", "Greater Swiss Mountain dog", "Bernese mountain dog", "Appenzeller", "EntleBucher", "boxer", "bull mastiff", "Tibetan mastiff", "French bulldog", "Great Dane", "Saint Bernard", "Eskimo dog", "malamute", "Siberian husky", "dalmatian", "affenpinscher", "basenji", "pug", "Leonberg", "Newfoundland", "Great Pyrenees", "Samoyed", "Pomeranian", "chow", "keeshond", "Brabancon griffon", "Pembroke", "Cardigan", "toy poodle", "miniature poodle", "standard poodle", "Mexican hairless", "timber wolf", "white wolf", "red wolf", "coyote", "dingo", "dhole", "African hunting dog", "hyena", "red fox", "kit fox", "Arctic fox", "grey fox", "tabby", "tiger cat", "Persian cat", "Siamese cat", "Egyptian cat", "cougar", "lynx", "leopard", "snow leopard", "jaguar", "lion", "tiger", "cheetah", "brown bear", "American black bear", "ice bear", "sloth bear", "mongoose", "meerkat", "tiger beetle", "ladybug", "ground beetle", "long-horned beetle", "leaf beetle", "dung beetle", "rhinoceros beetle", "weevil", "fly", "bee", "ant", "grasshopper", "cricket", "walking stick", "cockroach", "mantis", "cicada", "leafhopper", "lacewing", "dragonfly", "damselfly", "admiral", "ringlet", "monarch", "cabbage butterfly", "sulphur butterfly", "lycaenid", "starfish", "sea urchin", "sea cucumber", "wood rabbit", "hare", "Angora", "hamster", "porcupine", "fox squirrel", "marmot", "beaver", "guinea pig", "sorrel", "zebra", "hog", "wild boar", "warthog", "hippopotamus", "ox", "water buffalo", "bison", "ram", "bighorn", "ibex", "hartebeest", "impala", "gazelle", "Arabian camel", "llama", "weasel", "mink", "polecat", "black-footed ferret", "otter", "skunk", "badger", "armadillo", "three-toed sloth", "orangutan", "gorilla", "chimpanzee", "gibbon", "siamang", "guenon", "patas", "baboon", "macaque", "langur", "colobus", "proboscis monkey", "marmoset", "capuchin", "howler monkey", "titi", "spider monkey", "squirrel monkey", "Madagascar cat", "indri", "Indian elephant", "African elephant", "lesser panda", "giant panda", "barracouta", "eel", "coho", "rock beauty", "anemone fish", "sturgeon", "gar", "lionfish", "puffer", "abacus", "abaya", "academic gown", "accordion", "acoustic guitar", "aircraft carrier", "airliner", "airship", "altar", "ambulance", "amphibian", "analog clock", "apiary", "apron", "ashcan", "assault rifle", "backpack", "bakery", "balance beam", "balloon", "ballpoint", "Band Aid", "banjo", "bannister", "barbell", "barber chair", "barbershop", "barn", "barometer", "barrel", "barrow", "baseball", "basketball", "bassinet", "bassoon", "bathing cap", "bath towel", "bathtub", "beach wagon", "beacon", "beaker", "bearskin", "beer bottle", "beer glass", "bell cote", "bib", "bicycle-built-for-two", "bikini", "binder", "binoculars", "birdhouse", "boathouse", "bobsled", "bolo tie", "bonnet", "bookcase", "bookshop", "bottlecap", "bow", "bow tie", "brass", "brassiere", "breakwater", "breastplate", "broom", "bucket", "buckle", "bulletproof vest", "bullet train", "butcher shop", "cab", "caldron", "candle", "cannon", "canoe", "can opener", "cardigan", "car mirror", "carousel", "carpenter's kit", "carton", "car wheel", "cash machine", "cassette", "cassette player", "castle", "catamaran", "CD player", "cello", "cellular telephone", "chain", "chainlink fence", "chain mail", "chain saw", "chest", "chiffonier", "chime", "china cabinet", "Christmas stocking", "church", "cinema", "cleaver", "cliff dwelling", "cloak", "clog", "cocktail shaker", "coffee mug", "coffeepot", "coil", "combination lock", "computer keyboard", "confectionery", "container ship", "convertible", "corkscrew", "cornet", "cowboy boot", "cowboy hat", "cradle", "crane", "crash helmet", "crate", "crib", "Crock Pot", "croquet ball", "crutch", "cuirass", "dam", "desk", "desktop computer", "dial telephone", "diaper", "digital clock", "digital watch", "dining table", "dishrag", "dishwasher", "disk brake", "dock", "dogsled", "dome", "doormat", "drilling platform", "drum", "drumstick", "dumbbell", "Dutch oven", "electric fan", "electric guitar", "electric locomotive", "entertainment center", "envelope", "espresso maker", "face powder", "feather boa", "file", "fireboat", "fire engine", "fire screen", "flagpole", "flute", "folding chair", "football helmet", "forklift", "fountain", "fountain pen", "four-poster", "freight car", "French horn", "frying pan", "fur coat", "garbage truck", "gasmask", "gas pump", "goblet", "go-kart", "golf ball", "golfcart", "gondola", "gong", "gown", "grand piano", "greenhouse", "grille", "grocery store", "guillotine", "hair slide", "hair spray", "half track", "hammer", "hamper", "hand blower", "hand-held computer", "handkerchief", "hard disc", "harmonica", "harp", "harvester", "hatchet", "holster", "home theater", "honeycomb", "hook", "hoopskirt", "horizontal bar", "horse cart", "hourglass", "iPod", "iron", "jack-o'-lantern", "jean", "jeep", "jersey", "jigsaw puzzle", "jinrikisha", "joystick", "kimono", "knee pad", "knot", "lab coat", "ladle", "lampshade", "laptop", "lawn mower", "lens cap", "letter opener", "library", "lifeboat", "lighter", "limousine", "liner", "lipstick", "Loafer", "lotion", "loudspeaker", "loupe", "lumbermill", "magnetic compass", "mailbag", "mailbox", "maillot", "maillot", "manhole cover", "maraca", "marimba", "mask", "matchstick", "maypole", "maze", "measuring cup", "medicine chest", "megalith", "microphone", "microwave", "military uniform", "milk can", "minibus", "miniskirt", "minivan", "missile", "mitten", "mixing bowl", "mobile home", "Model T", "modem", "monastery", "monitor", "moped", "mortar", "mortarboard", "mosque", "mosquito net", "motor scooter", "mountain bike", "mountain tent", "mouse", "mousetrap", "moving van", "muzzle", "nail", "neck brace", "necklace", "nipple", "notebook", "obelisk", "oboe", "ocarina", "odometer", "oil filter", "organ", "oscilloscope", "overskirt", "oxcart", "oxygen mask", "packet", "paddle", "paddlewheel", "padlock", "paintbrush", "pajama", "palace", "panpipe", "paper towel", "parachute", "parallel bars", "park bench", "parking meter", "passenger car", "patio", "pay-phone", "pedestal", "pencil box", "pencil sharpener", "perfume", "Petri dish", "photocopier", "pick", "pickelhaube", "picket fence", "pickup", "pier", "piggy bank", "pill bottle", "pillow", "ping-pong ball", "pinwheel", "pirate", "pitcher", "plane", "planetarium", "plastic bag", "plate rack", "plow", "plunger", "Polaroid camera", "pole", "police van", "poncho", "pool table", "pop bottle", "pot", "potter's wheel", "power drill", "prayer rug", "printer", "prison", "projectile", "projector", "puck", "punching bag", "purse", "quill", "quilt", "racer", "racket", "radiator", "radio", "radio telescope", "rain barrel", "recreational vehicle", "reel", "reflex camera", "refrigerator", "remote control", "restaurant", "revolver", "rifle", "rocking chair", "rotisserie", "rubber eraser", "rugby ball", "rule", "running shoe", "safe", "safety pin", "saltshaker", "sandal", "sarong", "sax", "scabbard", "scale", "school bus", "schooner", "scoreboard", "screen", "screw", "screwdriver", "seat belt", "sewing machine", "shield", "shoe shop", "shoji", "shopping basket", "shopping cart", "shovel", "shower cap", "shower curtain", "ski", "ski mask", "sleeping bag", "slide rule", "sliding door", "slot", "snorkel", "snowmobile", "snowplow", "soap dispenser", "soccer ball", "sock", "solar dish", "sombrero", "soup bowl", "space bar", "space heater", "space shuttle", "spatula", "speedboat", "spider web", "spindle", "sports car", "spotlight", "stage", "steam locomotive", "steel arch bridge", "steel drum", "stethoscope", "stole", "stone wall", "stopwatch", "stove", "strainer", "streetcar", "stretcher", "studio couch", "stupa", "submarine", "suit", "sundial", "sunglass", "sunglasses", "sunscreen", "suspension bridge", "swab", "sweatshirt", "swimming trunks", "swing", "switch", "syringe", "table lamp", "tank", "tape player", "teapot", "teddy", "television", "tennis ball", "thatch", "theater curtain", "thimble", "thresher", "throne", "tile roof", "toaster", "tobacco shop", "toilet seat", "torch", "totem pole", "tow truck", "toyshop", "tractor", "trailer truck", "tray", "trench coat", "tricycle", "trimaran", "tripod", "triumphal arch", "trolleybus", "trombone", "tub", "turnstile", "typewriter keyboard", "umbrella", "unicycle", "upright", "vacuum", "vase", "vault", "velvet", "vending machine", "vestment", "viaduct", "violin", "volleyball", "waffle iron", "wall clock", "wallet", "wardrobe", "warplane", "washbasin", "washer", "water bottle", "water jug", "water tower", "whiskey jug", "whistle", "wig", "window screen", "window shade", "Windsor tie", "wine bottle", "wing", "wok", "wooden spoon", "wool", "worm fence", "wreck", "yawl", "yurt", "web site", "comic book", "crossword puzzle", "street sign", "traffic light", "book jacket", "menu", "plate", "guacamole", "consomme", "hot pot", "trifle", "ice cream", "ice lolly", "French loaf", "bagel", "pretzel", "cheeseburger", "hotdog", "mashed potato", "head cabbage", "broccoli", "cauliflower", "zucchini", "spaghetti squash", "acorn squash", "butternut squash", "cucumber", "artichoke", "bell pepper", "cardoon", "mushroom", "Granny Smith", "strawberry", "orange", "lemon", "fig", "pineapple", "banana", "jackfruit", "custard apple", "pomegranate", "hay", "carbonara", "chocolate sauce", "dough", "meat loaf", "pizza", "potpie", "burrito", "red wine", "espresso", "cup", "eggnog", "alp", "bubble", "cliff", "coral reef", "geyser", "lakeside", "promontory", "sandbar", "seashore", "valley", "volcano", "ballplayer", "groom", "scuba diver", "rapeseed", "daisy", "yellow lady's slipper", "corn", "acorn", "hip", "buckeye", "coral fungus", "agaric", "gyromitra", "stinkhorn", "earthstar", "hen-of-the-woods", "bolete", "ear", "toilet tissue"], "Receptive Field"=[{"V"=1, "H"=1}, {"V"=7, "H"=7}, {"V"=9, "H"=9}, {"V"=9, "H"=9}, {"V"=21, "H"=21}, {"V"=21, "H"=21}, {"V"=9, "H"=9}, {"V"=21, "H"=21}, {"V"=21, "H"=21}, {"V"=33, "H"=33}, {"V"=33, "H"=33}, {"V"=33, "H"=33}, {"V"=33, "H"=33}, {"V"=45, "H"=45}, {"V"=45, "H"=45}, {"V"=45, "H"=45}, {"V"=45, "H"=45}, {"V"=57, "H"=57}, {"V"=57, "H"=57}, {"V"=45, "H"=45}, {"V"=57, "H"=57}, {"V"=57, "H"=57}, {"V"=81, "H"=81}, {"V"=81, "H"=81}, {"V"=81, "H"=81}, {"V"=81, "H"=81}, {"V"=105, "H"=105}, {"V"=105, "H"=105}, {"V"=105, "H"=105}, {"V"=105, "H"=105}, {"V"=129, "H"=129}, {"V"=129, "H"=129}, {"V"=129, "H"=129}, {"V"=129, "H"=129}, {"V"=153, "H"=153}, {"V"=153, "H"=153}, {"V"=129, "H"=129}, {"V"=153, "H"=153}, {"V"=153, "H"=153}, {"V"=201, "H"=201}, {"V"=201, "H"=201}, {"V"=201, "H"=201}, {"V"=201, "H"=201}, {"V"=249, "H"=249}, {"V"=249, "H"=249}, {"V"=249, "H"=249}, {"V"=249, "H"=249}, {"V"=297, "H"=297}, {"V"=297, "H"=297}, {"V"=297, "H"=297}, {"V"=297, "H"=297}, {"V"=345, "H"=345}, {"V"=345, "H"=345}, {"V"=345, "H"=345}, {"V"=345, "H"=345}, {"V"=393, "H"=393}, {"V"=393, "H"=393}, {"V"=393, "H"=393}, {"V"=153, "H"=153}, {"V"=441, "H"=441}, {"V"=441, "H"=441}, {"V"=441, "H"=441}, {"V"=441, "H"=441}], "Loss_Type"=enum."MSE", "Loss_Cfg_Prms"=variant, "NNG_WS"={"NNG_WS_Mem"=refnum, "Max_WS_Size"=-1}}, "PCore_Device"=enum."GPU(CuLab)", "PatchCore_Init_CFG"={"BackBone"=enum."WRN_50_2_L2L3", "Out_Layers_Names"=[], "Patch_Size"=0}, "Coreset Params"={"Sampling_Ratio"=0.0, "Startd_idx"=0, "Random_Proj?"=FALSE, "Rnd. Proj. Params"={"Proj._Dim."=0, "Epsilon"=0.9, "Seed"=42}}, "MemBank_Data"={"MemBank"=variant, "MemBank Norm"=variant}} ("PCore_Instance"), "NN"=w18, "PatchCore_Init_CFG"=w13, "PCore_Device"=w14, "Dataset_Stats"=w31, "Coreset Params"=w12) -> (w15:T3)
      n14 = call "PatchCore_Set_Custom_Projection_Matrix.vi"("error in"=w21, "Out_Layers_Idx"=w11, "PCore_Instance in"=w15) -> ("error out"=w20:errorcluster, "PCore_Instance out"=w19:T3)  [unwired: 7 in]
      n15 = call "Get_Exec_Time.vim"("T(n-1)"=w24, "error in (no error)"=w20) -> ("error out"=w27:errorcluster, "dT"=w26:dbl)  [unwired: 5 in, 1 out]
    }
    frame Error {
    }
  }
  "error out" <- w7
  "dT" <- w6
  "PCore_Instance out" <- w3
